vi "Test Set Row Values Append Bool.vi"(11 "Test Case In":refnum<class "Test Open Xml.lvclass">) -> (0 "error out":errorcluster, 3 "Test Case Out":refnum<class "Test Open Xml.lvclass">)   [LabVIEW 2020, in "Test Open Xml.lvclass"]
uses:
  Test Open Xml.lvclass
  <vilib>/Astemes/LUnit/Test Case.lvclass
  Source/Open Xml.lvlib
  Source/Cell DataType.ctl
panel:
  out "Numeric":dbl
  # "200 - 3.6sec"
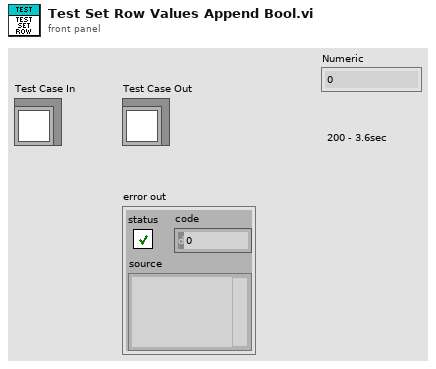
[diagram p1: front panel]
types:
  T1 = typedef "Open Xml.lvlib/Cell DataType.ctl" = enum16{"Void", "Boolean", "Number", "Error", "SharedString", "String", "InlineString", "Date"}
  T2 = cluster{"Number":dbl, "String":string, "Boolean":bool, "Time Stamp":timestamp, "Error":errorcluster}[]
  T3 = cluster{"Number":dbl, "String":string, "Boolean":bool, "Time Stamp":timestamp, "Error":errorcluster}
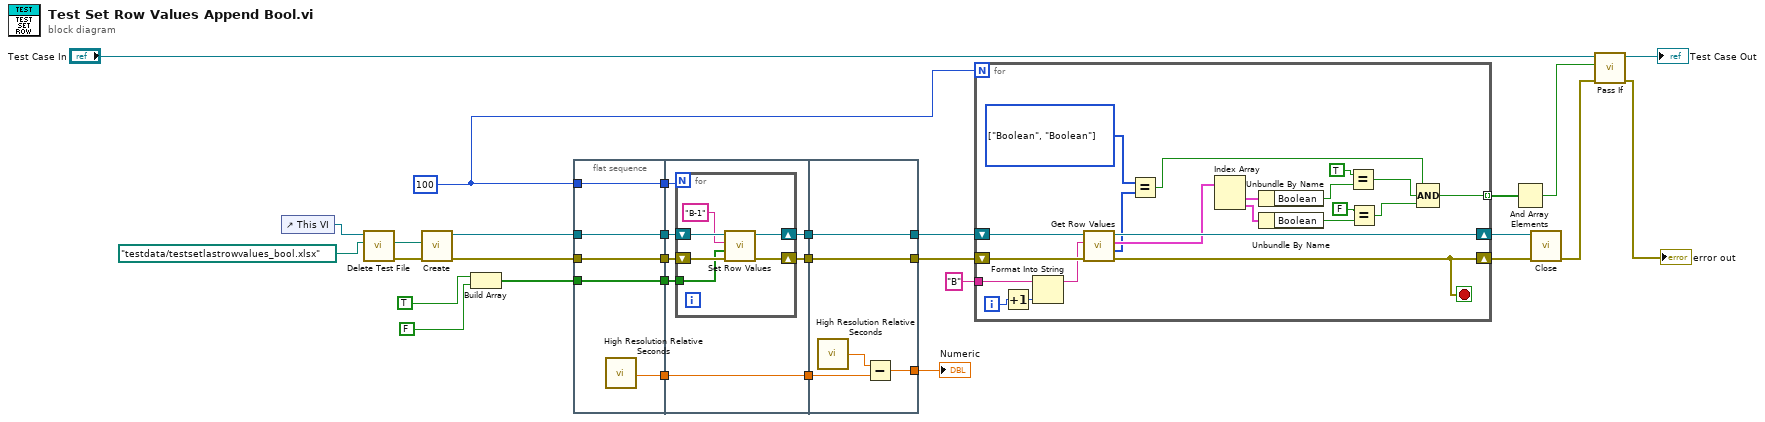
[diagram p0: block diagram]
diagram:
  w12 = 100
  n1 = control-ref of="This VI"() -> (w15:refnum<vi>)
  n2 = call "Delete Test File.vi"("name or relative path"=path "testdata/testsetlastrowvalues_bool.xlsx", "VI in"=w15) -> ("error out"=w16:errorcluster, "deleted path"=w13:path)  [unwired: 8 in]
  n3 = call "Create.vi"("error in"=w16, "Path"=w13) -> ("error out"=w26:errorcluster, "SpreadsheetDoc"=w27:refnum<k24>)  [unwired: 8 in]
  n4 = Build Array(TRUE, FALSE) -> (w20:bool[])
  n5 = flat-sequence {
    tunnel: w12 -> [w32]
    tunnel: w20 -> [w33]
    tunnel: w26 -> [w34]
    tunnel: w27 -> [w35]
    tunnel: [w35] -> w9
    tunnel: [w34] -> w8
    tunnel: [w33] -> w7
    tunnel: [w32] -> w6
    tunnel: [w31] -> w3
    tunnel: w9 -> [w42]
    tunnel: w8 -> [w41]
    tunnel: w7 -> [w38]
    tunnel: w6 -> [w37]
    tunnel: [w40] -> w5
    tunnel: [w39] -> w4
    tunnel: w3 -> [w36]
    tunnel: [w36] -> w2
    tunnel: [w52] -> w22
    tunnel: [w53] -> w23
    tunnel: w5 -> [w53]
    tunnel: w4 -> [w52]
    tunnel: w2 -> [w50]
    tunnel: [w49] -> w1
    frame #0 {
      n6 = call <vilib>:"High Resolution Relative Seconds.vi"() -> ("relative seconds"=w31:dbl)
    }
    frame #1 {
      n7 = for {
        N: w37 -> [_]
        tunnel: w38 -> [w43]
        shift-right: [w45] -> w39
        shift-left: w42 -> [w48]
        shift-right: [w46] -> w40
        shift-left: w41 -> [w47]
        n8 = call "Set Row Values.vi"("error in"=w47, "Values"=w43, "Cell Address"="B-1", "SpreadsheetDoc"=w48) -> ("error out"=w46:errorcluster, "SpreadsheetDoc out"=w45:refnum<k24>)  [unwired: 6 in]
      }
    }
    frame #2 {
      n9 = call <vilib>:"High Resolution Relative Seconds.vi"() -> ("relative seconds"=w51:dbl)
      n10 = Subtract(x=w51, y=w50) -> (x-y=w49:dbl)
    }
  }
  n11 = for {
    N: w12 -> [_]
    tunnel: "B" ("Cell Address") -> [w72]
    shift-right: [w54] -> w24
    shift-left: w23 -> [w74]
    shift-right: [w71] -> w19
    shift-left: w22 -> [w73]
    tunnel: [w55] -> w11 mode=indexing
    i -> [w69]
    stop <- w54 stop-if-true
    w67 = T1[] [enum."Boolean", enum."Boolean"] items=["Void", "Boolean", "Number", "Error", "SharedString", "String", "InlineString", "Date"] ("x")
    n12 = Increment(x=w69) -> (x+1=w68:i32)
    n13 = Format Into String(initial string=w72, w68) -> (resulting string=w70:string)  [unwired: 2 in, 1 out]
    n14 = call "Get Row Values.vi"("error in"=w74, "Row Address"=w70, "SpreadsheetDoc in"=w73) -> ("error out"=w54:errorcluster, "Types"=w59:T1[], "Cell Values"=w66:T2, "SpreadsheetDoc out"=w71:refnum<k24>)  [unwired: 5 in]
    n15 = Equal?(x=w67, y=w59) -> (x = y?=w56:bool)
    n16 = Index Array(array=w66) -> (element #1=w65:T3, element #2=w64:T3)  [unwired: 2 in]
    n17 = Unbundle By Name(w65) -> ("Boolean"=w61:bool)
    n18 = Unbundle By Name(w64) -> ("Boolean"=w63:bool)
    n19 = Equal?(x=TRUE, y=w61) -> (x = y?=w57:bool)
    n20 = Equal?(x=FALSE, y=w63) -> (x = y?=w58:bool)
    n21 = Compound Arithmetic op=AND(w56, w57, w58) -> (w55:bool)
  }
  n22 = And Array Elements(Boolean array=w11) -> (logical AND=w10:bool)
  n23 = call "Close.vi"("error in"=w24, "SpreadsheetDoc"=w19) -> ("error out"=w25:errorcluster)  [unwired: 9 in]
  n24 = call <vilib>:"Pass If.vi"("error in (no error)"=w25, "Pass?"=w10, "LUnit Test Case In"="Test Case In") -> ("error out"=→"error out":errorcluster, "LUnit Test Case Out"=→"Test Case Out":refnum<class "Test Open Xml.lvclass">)  [unwired: 7 in]
  "Numeric" <- w1
